vi "Set Current.vi"(8 "error in":errorcluster, 10 "%":dbl, 11 "4-20mA Out Settings In":T1) -> (0 "error out":errorcluster, 1 "Connection Error":bool, 3 "4-20mA Out Settings Out":T1)   [LabVIEW 2018, in "Pressure Regulator Library.lvlib"]
uses:
  Pressure Regulator Library.lvlib
  Pressure Regulator Device Settings.ctl
  <vilib>/Utility/error.llb/DialogType.ctl
  <vilib>/DAQmx/write.llb/DAQmx Write (Analog DBL 1Chan 1Samp).vi
  <vilib>/DAQmx/miscellaneous.llb/DAQmx Fill In Error Info.vi
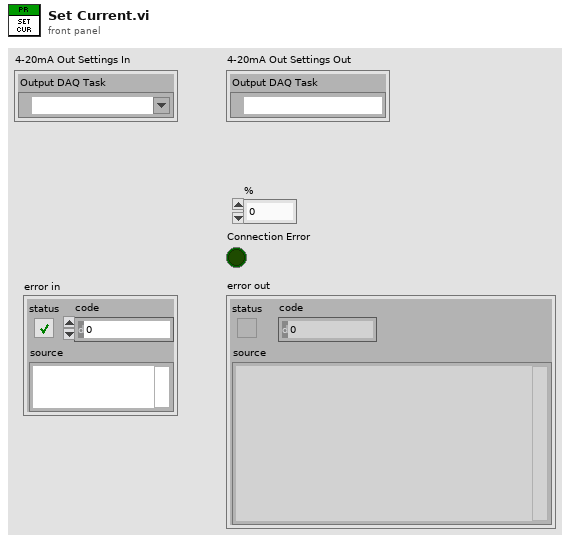
[diagram p1: front panel]
types:
  T1 = typedef "Pressure Regulator Library.lvlib/Pressure Regulator Device Settings.ctl" = cluster{"Output DAQ Task":refnum<k21>}
  T2 = typedef "DialogType.ctl" = u16
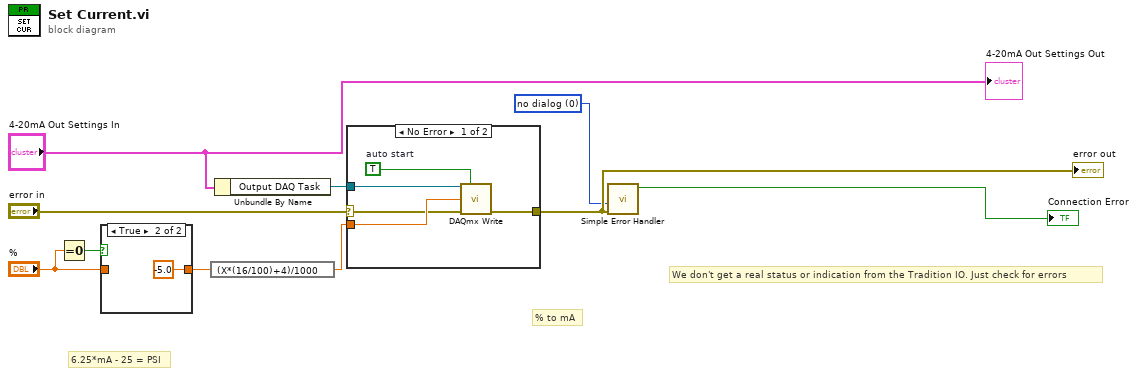
[diagram p0: block diagram]
diagram:
  w4 = T2 0 items=["no dialog", "OK message", "continue or stop message", "OK message + warnings", "continue/stop + warnings"] ("type of dialog (OK msg:1)")
  # "6.25*mA - 25 = PSI"
  # "We don't get a real status or indication from the Tradition IO. Just check for errors"
  # "% to mA"
  n1 = Equal To 0?(x="%") -> (x = 0?=w3:bool)
  n2 = case shown="True" w3 {
    tunnel: "%" -> [w11 _]
    tunnel: [w11 -5.0] -> w1
    frame False {
    }
    frame True {
    }
  }
  n3 = expression code="(X*(16/100)+4)/1000"(w1) -> (w10:dbl)
  n4 = Unbundle By Name("4-20mA Out Settings In") -> ("Output DAQ Task"=w8:refnum<k21>)
  n5 = case shown="No Error" "error in" {
    selector: "error in" -> [w13 w18]
    tunnel: w10 -> [w14 _]
    tunnel: w8 -> [w17 _]
    tunnel: [w15 w18] -> w5
    frame No Error {
      w16 = TRUE  # auto start
      n6 = call-poly <vilib>:"DAQmx Write.vi"("task/channels in"=w17, "auto start"=w16, "data"=w14, "error in"=w13) -> ("error out"=w15:errorcluster)  [unwired: 9 in, 2 out]
    }
    frame Error {
    }
  }
  "error out" <- w5
  n7 = call <vilib>:"Simple Error Handler.vi"("type of dialog (OK msg:1)"=w4, "error in (no error)"=w5) -> ("error?"=→"Connection Error":bool)  [unwired: 3 in, 4 out]
  "4-20mA Out Settings Out" <- "4-20mA Out Settings In"
